vi "Write Element of CellData.vi"(8 "error in (no error)":errorcluster, 9 "PAS Cell Data.lvclass":refnum<class "PAS Cell Data.lvclass">, 10 "index":i32, 11 "PAS Data in":refnum<class "PAS Data.lvclass">) -> (0 "error out":errorcluster, 3 "PAS Data out":refnum<class "PAS Data.lvclass">)   [LabVIEW 2015, in "PAS Data.lvclass"]
uses:
  PAS Data.lvclass
  Cell/PAS Cell Data.lvclass
  PAS Data.lvclass/PAS Data.ctl
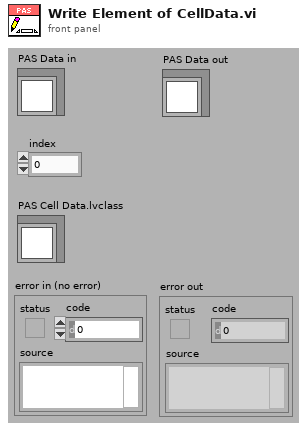
[diagram p1: front panel]
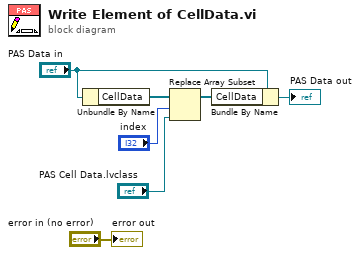
[diagram p0: block diagram]
diagram:
  n1 = Unbundle By Name("PAS Data in") -> ("CellData"=w3:refnum<class "PAS Cell Data.lvclass">[])
  n2 = Replace Array Subset(array=w3, new element="PAS Cell Data.lvclass", index="index") -> (w2:refnum<class "PAS Cell Data.lvclass">[])
  n3 = Bundle By Name(cluster="PAS Data in", "CellData"=w2) -> (→"PAS Data out":refnum<class "PAS Data.lvclass">)
  "error out" <- "error in (no error)"
